vi "Main.vi"() -> ()   [LabVIEW 2025, in "phlair-busch-can-bus.lvlib"]
doc: "This example demonstrates sending automatically converted values of signals using an NI-XNET Signal Output session. \n\nThis examples is made to be run against the CAN Signal Input Single Point (Session) example, assuming you have a properly terminated CAN cable connected to two CAN ports.\n\nIf you do not have any database aliases on your system, the example will automatically load the nixnet_example database."
uses:
  phlair-busch-can-bus.lvlib
  <vilib>/xnet/xnet.llb/XNET Write (Signal Single-point).vi
  <vilib>/xnet/xnet.llb/XNET Read (Frame CAN).vi
  <vilib>/xnet/xnet.llb/XNET Frame Type CAN.ctl
  <vilib>/xnet/xnet.llb/XNET Frame CAN.ctl
  CAN Frame Sessions.ctl
  DilicoControls.ctl
panel:
  out "CAN Frame Output (only query)":T1[](array[typedef]) {"payload" format="%x"; "timestamp" format="%<%.7X\n%x>T"; "type" items=["CAN Data"=0, "CAN Remote"=1, "CAN Bus Error"=2, "CAN 2.0 Data"=8, "CAN FD Data"=16, "CAN FD+BRS Data"=24, "J1939 Data"=192, "Delay"=224, "Log Trigger"=225, "Start Trigger"=226]; "identifier" format="%x"}
  in  "Query":bool
  out "CVM":cluster{i32[], dbl[]}[](graph)
  out "Cell(s) UV":string
  out "Cell(s) OV":string
  out "Plot(s)":i32
  out "Average":dbl format="%#_6f"
  out "Min":dbl
  out "Max":dbl
  out "Stack V":dbl
  in  "CAN Frame Sessions":T3={"Session_Control"="Sess_Control", "Session_Params"="Sess_Params", "Session_Actuals"="Sess_Actuals", "Session_Acknowledge"="Sess_Ack", "Session_H2_Sensor"="H2_Sensor_Session", "Session_DILICO_MeasurementRequest"="Session_DILICO_MeasurementRequest", "Session_DILICO_Voltages"="Session_DILICO_Voltages"}
  in  "Dilico Measurement Controls":T4={"Number of cells"=10, "Wait time [ms]"=2.0, "UnderVoltage Limit [mV]"=1, "OverVoltage Limit [mV]"=10} {"OverVoltage Limit [mV]" max=5000 step=1; "Wait time [ms]" min=0 max=25.5; "UnderVoltage Limit [mV]" max=5000 step=1}
  out "Number of Frames Received":i32
  out "CAN Frame Input":T1[](array[typedef]) {"payload" format="%x"; "timestamp" format="%<%.7X\n%x>T"; "type" items=["CAN Data"=0, "CAN Remote"=1, "CAN Bus Error"=2, "CAN 2.0 Data"=8, "CAN FD Data"=16, "CAN FD+BRS Data"=24, "J1939 Data"=192, "Delay"=224, "Log Trigger"=225, "Start Trigger"=226]; "identifier" format="%x"}
  out "data":u8[](array[numeric])=[10, 10, 0, 1, 0, 2] format="%.0x"
  in  "Set Measurement":bool
  in  "stop":bool
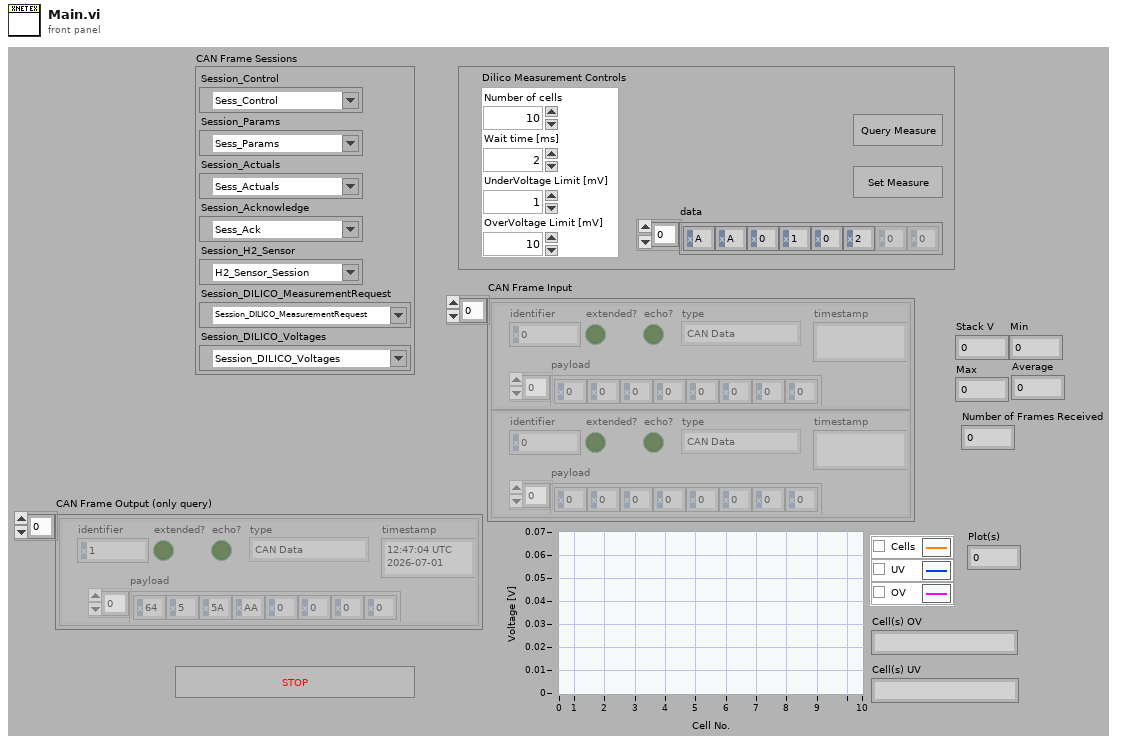
[diagram p1: front panel]
types:
  T1 = typedef "XNET Frame CAN.ctl" = cluster{"timestamp":timestamp, "payload":u8[], "identifier":u32, "type":T2, "extended?":bool, "echo?":bool}
  T2 = typedef "XNET Frame Type CAN.ctl" = u8
  T3 = typedef "phlair-busch-can-bus.lvlib/CAN Frame Sessions.ctl" = cluster{"Session_Control":refnum<k21>, "Session_Params":refnum<k21>, "Session_Actuals":refnum<k21>, "Session_Acknowledge":refnum<k21>, "Session_H2_Sensor":refnum<k21>, "Session_DILICO_MeasurementRequest":refnum<k21>, "Session_DILICO_Voltages":refnum<k21>}
  T4 = typedef "phlair-busch-can-bus.lvlib/DilicoControls.ctl" = cluster{"Number of cells":u8, "Wait time [ms]":sgl, "UnderVoltage Limit [mV]":u16, "OverVoltage Limit [mV]":u16}
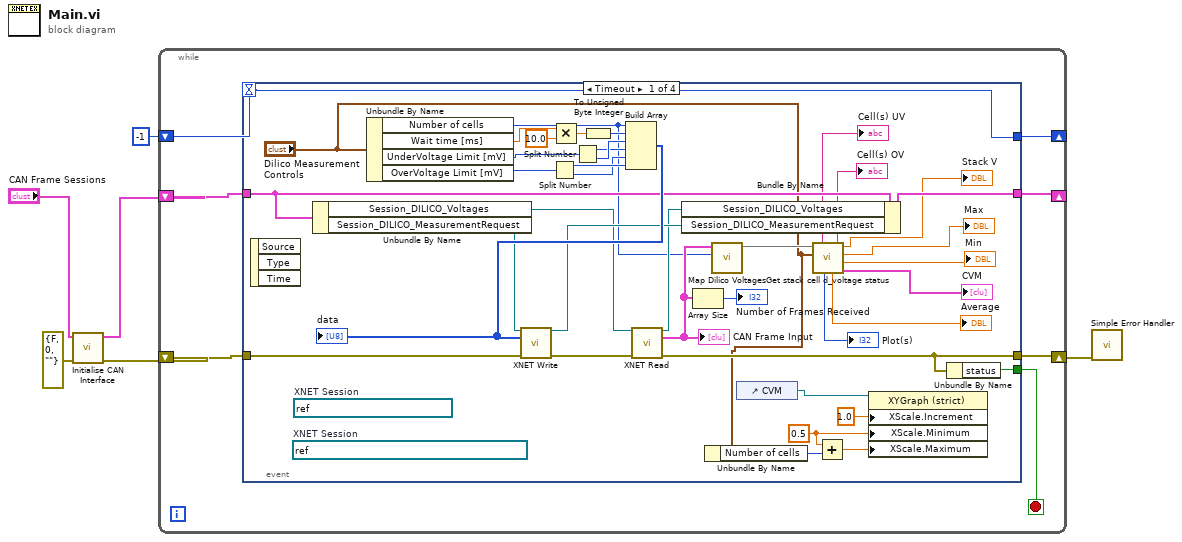
[diagram p0: block diagram]
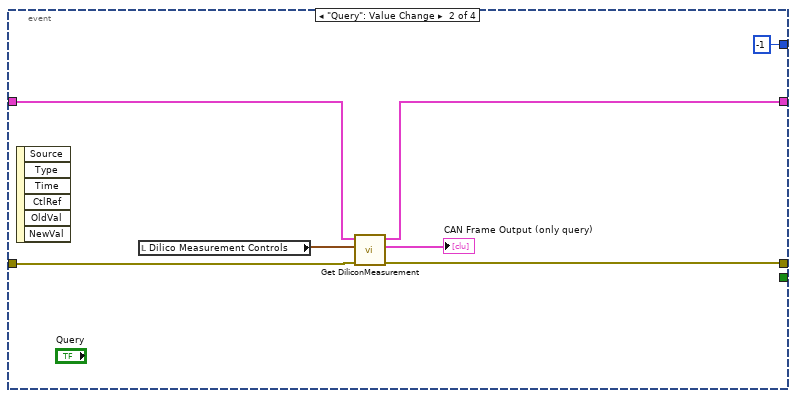
[diagram p2: hidden frame]
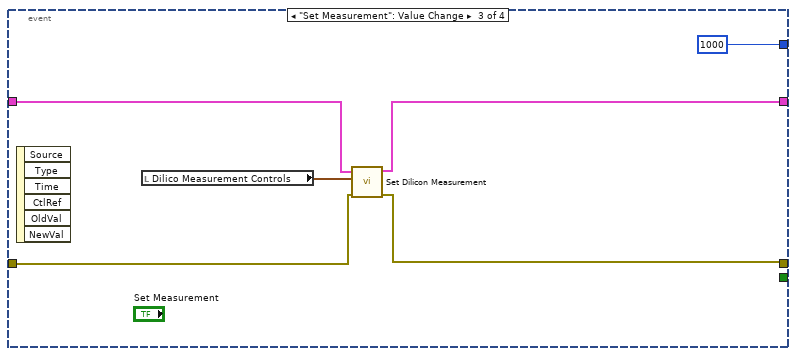
[diagram p3: hidden frame]
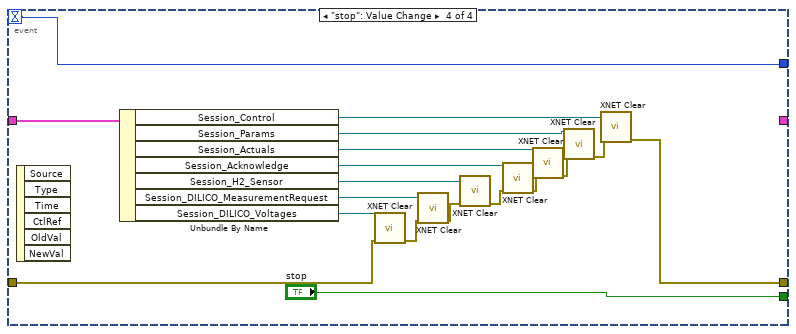
[diagram p4: hidden frame]
diagram:
  n1 = call "Initialise CAN Interface.vi"("error in (no error)"=errorcluster {"status"=FALSE, "code"=0, "source"=""}, "CAN Frame Sessions"="CAN Frame Sessions") -> ("error out"=w5:errorcluster, "output cluster"=w2:T3)  [unwired: 8 in]
  n2 = while {
    shift-right: [w13] -> w6
    shift-left: w5 -> [w11]
    shift-right: [w9] -> _
    shift-left: w2 -> [w10]
    shift-right: [w8] -> _
    shift-left: -1 -> [w7]
    stop <- w12 stop-if-true
    n3 = event shown="[0] Timeout" {
      selector: _ -> [_ _ _ _]
      dyn-events: _ -> [_ _ _ _]
      timeout: w7 -> [w14 _ _ w68]
      tunnel: [w50 w59 w65 w69] -> w13
      tunnel: [w53 _ _ "stop"] -> w12
      tunnel: w11 -> [w52 w60 w66 w76]
      tunnel: w10 -> [w37 w57 w64 w67]
      tunnel: [w36 w58 w63 _] -> w9
      tunnel: [w14 -1 1000 w68] -> w8
      event Timeout {
        w23 = 0.5 ("X Scale.Range:Minimum")
        (unwired) refnum<k21> "Session_DILOCO_MeasurementRequest"  # XNET Session
        (unwired) refnum<k21> "Session_DILICO_Voltages"  # XNET Session
        n4 = event-data() -> ()  [unwired: 1 in, 3 out]
        n5 = Unbundle By Name(w37) -> ("Session_DILICO_Voltages"=w15:refnum<k21>, "Session_DILICO_MeasurementRequest"=w16:refnum<k21>)
        n6 = Unbundle By Name("Dilico Measurement Controls") -> ("Number of cells"=w33:u8, "Wait time [ms]"=w40:sgl, "UnderVoltage Limit [mV]"=w45:u16, "OverVoltage Limit [mV]"=w41:u16)
        n7 = Split Number(x=w41) -> (hi(x)=w42:u8, lo(x)=w38:u8)
        n8 = Multiply(x=w40, y=10.0) -> (x*y=w47:dbl)
        n9 = Split Number(x=w45) -> (hi(x)=w43:u8, lo(x)=w44:u8)
        n10 = To Unsigned Byte Integer(number=w47) -> (unsigned 8bit integer=w46:u8)
        n11 = Build Array(w33, w46, w44, w43, w38, w42) -> (w39:u8[])
        "data" <- w39
        n12 = call-poly <vilib>:"XNET Write.vi"("session in"=w16, "data"=w39, "error in (no error)"=w52) -> ("session out"=w35:refnum<k21>, "error out"=w17:errorcluster)  [unwired: 11 out]
        n13 = call-poly <vilib>:"XNET Read.vi"("session in"=w15, "error in (no error)"=w17) -> ("session out"=w34:refnum<k21>, "data"=w49:T1[], "error out"=w50:errorcluster)  [unwired: 11 out]
        "CAN Frame Input" <- w49
        n14 = Bundle By Name(cluster=w37, "Session_DILICO_Voltages"=w34, "Session_DILICO_MeasurementRequest"=w35) -> (w36:T3)
        n15 = Array Size(array=w49) -> (size(s)=→"Number of Frames Received":i32)
        n16 = Unbundle By Name("Dilico Measurement Controls") -> ("Number of cells"=w18:u8)
        n17 = call "Map Dilico Voltages.vi"("#Cell Request"=w33, "CAN Frame Input"=w49) -> ("Dilico Values"=w32:map{string, dbl})  [unwired: 9 in]
        n18 = control-ref of="CVM"() -> (w21:refnum<vi>)
        n19 = call "Get stack cell d_voltage status.vi"("Dilico Measurement Controls"="Dilico Measurement Controls", "Status Map"=w32) -> ("CVM"=→"CVM":cluster{i32[], dbl[]}[], "Min"=→"Min":dbl, "Max"=→"Max":dbl, "Sum Stack V"=→"Stack V":dbl, "Average"=→"Average":dbl, "Cell(s) OV"=→"Cell(s) OV":string, "Plot(s)"=→"Plot(s)":i32, "Cell(s) UV"=→"Cell(s) UV":string)  [unwired: 2 in]
        n20 = Add(x=w23, y=w18) -> (x+y=w22:dbl)
        n21 = property class="XYGraph (strict)"(reference=w21, "XScale.Increment"=1.0 ("X Scale.Range:Increment"), "XScale.Minimum"=w23, "XScale.Maximum"=w22) -> ()  [unwired: 1 in, 2 out]
        n22 = Unbundle By Name(w50) -> ("status"=w53:bool)
      }
      event "Query": Value Change {
        n23 = event-data() -> ()  [unwired: 1 in, 6 out]
        n24 = local read "Dilico Measurement Controls"() -> (w56:T4)
        n25 = call "Get DiliconMeasurement.vi"("error in (no error)"=w60, "Dilico Measurement Controls"=w56, "input cluster"=w57) -> ("error out"=w59:errorcluster, "CAN Frame Output"=→"CAN Frame Output (only query)":T1[], "output cluster"=w58:T3)  [unwired: 6 in]
      }
      event "Set Measurement": Value Change {
        n26 = event-data() -> ()  [unwired: 1 in, 6 out]
        n27 = local read "Dilico Measurement Controls"() -> (w62:T4)
        n28 = call "Set Dilicon Measurement.vi"("error in (no error)"=w66, "Dilico Measurement Controls"=w62, "input cluster"=w64) -> ("error out"=w65:errorcluster, "output cluster"=w63:T3)  [unwired: 7 in]
      }
      event "stop": Value Change {
        n29 = event-data() -> ()  [unwired: 1 in, 6 out]
        n30 = Unbundle By Name(w67) -> ("Session_Control"=w83:refnum<k21>, "Session_Params"=w78:refnum<k21>, "Session_Actuals"=w77:refnum<k21>, "Session_Acknowledge"=w79:refnum<k21>, "Session_H2_Sensor"=w80:refnum<k21>, "Session_DILICO_MeasurementRequest"=w81:refnum<k21>, "Session_DILICO_Voltages"=w82:refnum<k21>)
        n31 = call <vilib>:"XNET Clear.vi"("session in"=w82, "error in (no error)"=w76) -> ("error out"=w75:errorcluster)  [unwired: 13 in]
        n32 = call <vilib>:"XNET Clear.vi"("session in"=w81, "error in (no error)"=w75) -> ("error out"=w74:errorcluster)  [unwired: 13 in]
        n33 = call <vilib>:"XNET Clear.vi"("session in"=w80, "error in (no error)"=w74) -> ("error out"=w73:errorcluster)  [unwired: 13 in]
        n34 = call <vilib>:"XNET Clear.vi"("session in"=w79, "error in (no error)"=w73) -> ("error out"=w72:errorcluster)  [unwired: 13 in]
        n35 = call <vilib>:"XNET Clear.vi"("session in"=w77, "error in (no error)"=w72) -> ("error out"=w71:errorcluster)  [unwired: 13 in]
        n36 = call <vilib>:"XNET Clear.vi"("session in"=w78, "error in (no error)"=w71) -> ("error out"=w70:errorcluster)  [unwired: 13 in]
        n37 = call <vilib>:"XNET Clear.vi"("session in"=w83, "error in (no error)"=w70) -> ("error out"=w69:errorcluster)  [unwired: 13 in]
      }
    }
  }
  n38 = call <vilib>:"Simple Error Handler.vi"("error in (no error)"=w6) -> ()  [unwired: 1 in, 8 out]
